vi "generate multiple MCL offset.vi"(3 "Offset array":dbl[](array[numeric]), 4 "offset file step size":dbl, 5 "MCL offset scanning range (V)":T2={"Min X"=5.0, "Max X"=10.0, "Min Y"=5.0, "Max Y"=10.0, "Scan increment"=5.0}, 6 "Corrections":dbl[](array[numeric])) -> (0 "B_X mean out":dbl[](array[numeric]), 1 "A_X mean out":dbl[](array[numeric]), 2 "Output array":T1(array[cluster]))   [LabVIEW 2014]
panel:
  # "Values along Y axis"
  # "Value along \nx axis"
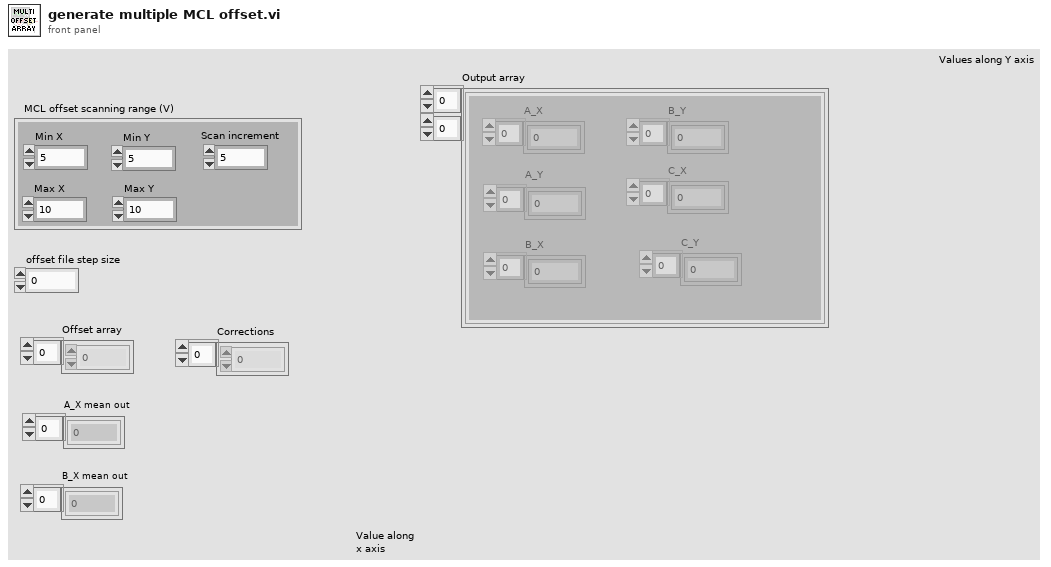
[diagram p1: front panel]
types:
  T1 = cluster{"A_X":dbl[], "A_Y":dbl[], "B_X":dbl[], "B_Y":dbl[], "C_X":dbl[], "C_Y":dbl[]}[][]
  T2 = cluster{"Min X":dbl, "Max X":dbl, "Min Y":dbl, "Max Y":dbl, "Scan increment":dbl}
  T3 = cluster{dbl[], dbl[], dbl[], dbl[], dbl[], dbl[]}
  T4 = cluster{dbl[], dbl[], dbl[], dbl[], dbl[], dbl[]}[][]
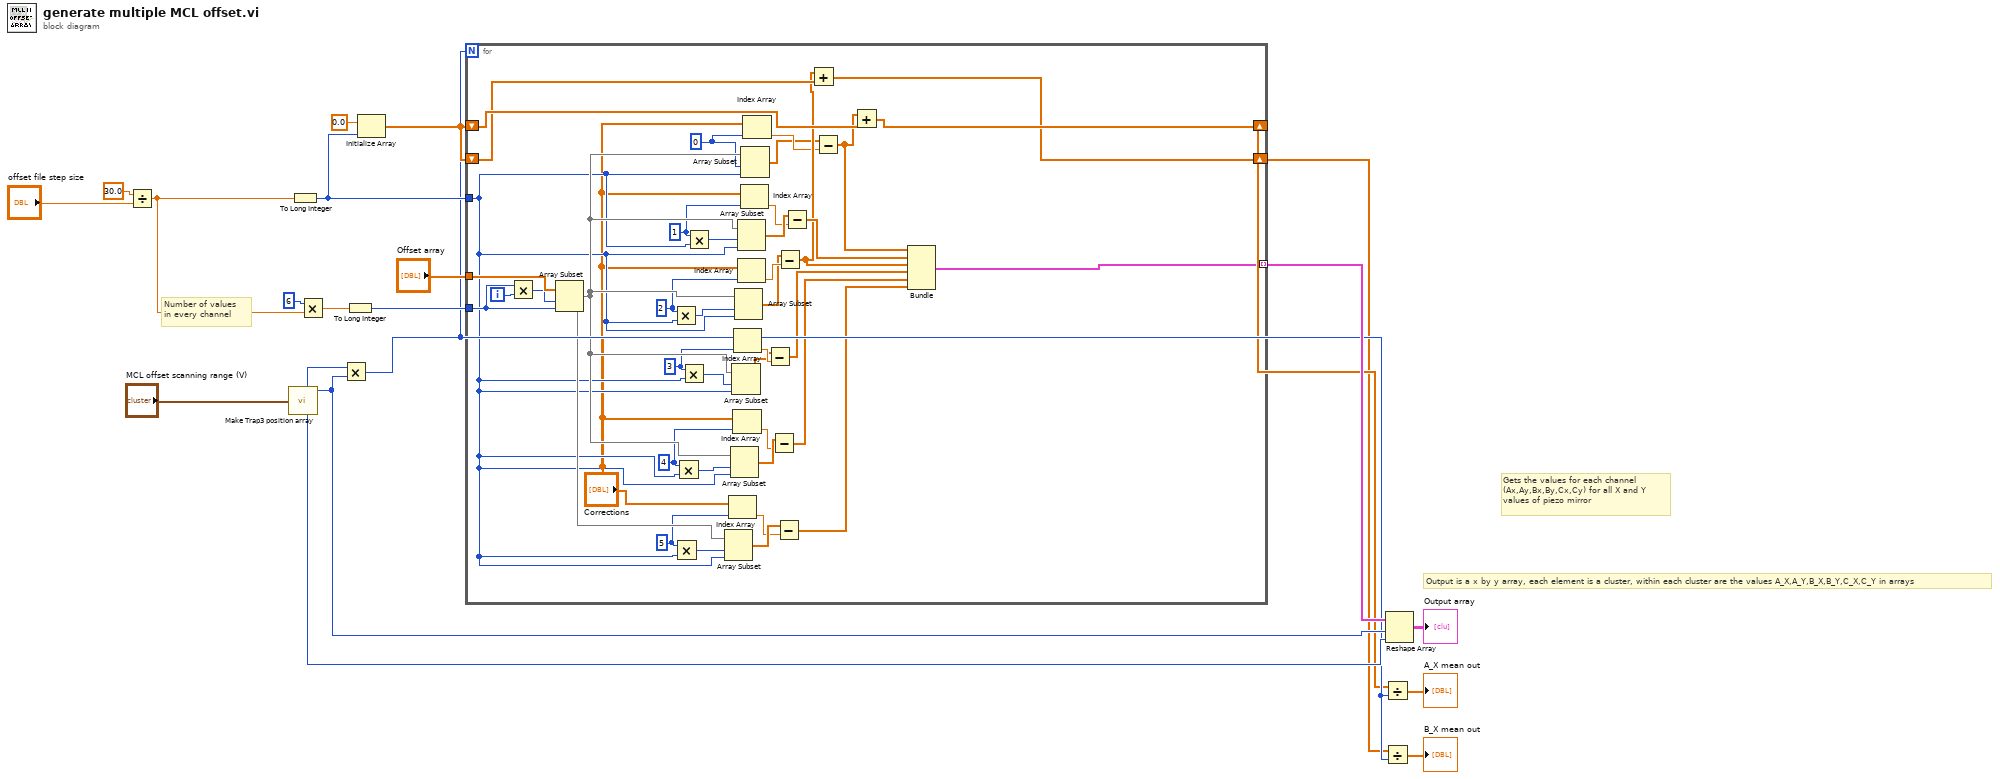
[diagram p0: block diagram]
diagram:
  # "Output is a x by y array, each element is a cluster, within each cluster are the values A_X,A_Y,B_X,B_Y,C_X,C_Y in arrays"
  # "Gets the values for each channel\n(Ax,Ay,Bx,By,Cx,Cy) for all X and Y \nvalues of piezo mirror"
  # "Number of values\nin every channel"
  n1 = Divide(x=30.0, y="offset file step size") -> (x/y=w14:dbl)
  n2 = call "Make Trap3 position array.vi"("MCL offset scanning range (V)"="MCL offset scanning range (V)") -> ("X Data points"=w12:u64, "Y data points"=w11:u64)  [unwired: 3 out]
  n3 = To Long Integer(number=w14) -> (32bit integer=w8:i32)
  n4 = Multiply(x=6, y=w14) -> (x*y=w17:dbl)
  n5 = Multiply(x=w11, y=w12) -> (x*y=w5:u64)
  n6 = To Long Integer(number=w17) -> (32bit integer=w16:i32)
  n7 = Initialize Array(0.0, w8) -> (w6:dbl[])
  n8 = for {
    N: w5 -> [_]
    tunnel: "Offset array" -> [w61]
    tunnel: w16 -> [w59]
    tunnel: w8 -> [w47]
    tunnel: [w52] -> w13 mode=indexing
    shift-right: [w50] -> w4
    shift-left: w6 -> [w51]
    shift-right: [w48] -> w3
    shift-left: w6 -> [w49]
    i -> [w60]
    w30 = 1
    w45 = 5
    w41 = 4
    w37 = 3
    w32 = 2
    w25 = 0
    n9 = Multiply(x=w59, y=w60) -> (x*y=w58:i32)
    n10 = Array Subset(array=w61, index=w58, length=w59) -> (w57:dbl[])
    n11 = Multiply(x=w32, y=w47) -> (x*y=w54:i32)
    n12 = Multiply(x=w45, y=w47) -> (x*y=w55:i32)
    n13 = Multiply(x=w41, y=w47) -> (x*y=w56:i32)
    n14 = Multiply(x=w37, y=w47) -> (x*y=w53:i32)
    n15 = Multiply(x=w30, y=w47) -> (x*y=w46:i32)
    n16 = Array Subset(array=w57, index=w55, length=w47) -> (w44:dbl[])
    n17 = Index Array(array="Corrections", index=w45) -> (element=w43:dbl)
    n18 = Array Subset(array=w57, index=w56, length=w47) -> (w40:dbl[])
    n19 = Array Subset(array=w57, index=w53, length=w47) -> (w35:dbl[])
    n20 = Index Array(array="Corrections", index=w41) -> (element=w39:dbl)
    n21 = Index Array(array="Corrections", index=w37) -> (element=w36:dbl)
    n22 = Array Subset(array=w57, index=w54, length=w47) -> (w31:dbl[])
    n23 = Array Subset(array=w57, index=w46, length=w47) -> (w29:dbl[])
    n24 = Index Array(array="Corrections", index=w32) -> (element=w33:dbl)
    n25 = Index Array(array="Corrections", index=w30) -> (element=w28:dbl)
    n26 = Array Subset(array=w57, index=w25, length=w47) -> (w22:dbl[])
    n27 = Index Array(array="Corrections", index=w25) -> (element=w23:dbl)
    n28 = Subtract(x=w35, y=w36) -> (x-y=w34:dbl[])
    n29 = Subtract(x=w40, y=w39) -> (x-y=w38:dbl[])
    n30 = Subtract(x=w44, y=w43) -> (x-y=w42:dbl[])
    n31 = Subtract(x=w31, y=w33) -> (x-y=w26:dbl[])
    n32 = Subtract(x=w29, y=w28) -> (x-y=w27:dbl[])
    n33 = Add(x=w26, y=w49) -> (x+y=w48:dbl[])
    n34 = Subtract(x=w22, y=w23) -> (x-y=w21:dbl[])
    n35 = Add(x=w21, y=w51) -> (x+y=w50:dbl[])
    n36 = Bundle(w21, w27, w26, w34, w38, w42) -> (w52:T3)  [unwired: 1 in]
  }
  n37 = Divide(x=w4, y=w5) -> (x/y=→"A_X mean out":dbl[])
  n38 = Divide(x=w3, y=w5) -> (x/y=→"B_X mean out":dbl[])
  n39 = Reshape Array(w13, w12, w11) -> (→"Output array":T4)
